vi "EquiRipple Filter Design - DFD.vi"() -> ()   [LabVIEW 2023]
doc: "Demonstrates how to design an Equi-Ripple FIR filter using VIs in the LabVIEW Digital Filter Design Toolkit. \n\nAs you change the Filter Type, experiment with the parameters for that filter type and observe their effect on the magnitude and phase responses."
uses:
  <vilib>/addons/Digital Filter Design/_Objects.llb/DFD Phase Setting.ctl
  <vilib>/addons/Digital Filter Design/Analysis.llb/DFD Plot Freq Response (Linear-Spaced).vi
  <vilib>/addons/Digital Filter Design/NI_DigFilterLicensed.lvlib
panel:
  out "Error message":string
  out "?":string="dB"
  in  "sampling rate":dbl=1000.0 format="%0.2f"
  in  "Display":bool=TRUE
  in  "Bandstop params":T1={"low pass frequency"=100.0, "high pass frequency"=400.0, "low stop frequency"=200.0, "high stop frequency"=300.0} {"high stop frequency" format="%0.2f"; "low stop frequency" format="%0.2f"; "high pass frequency" format="%0.2f"; "low pass frequency" format="%0.2f"}
  in  "Bandpass params":T1={"low pass frequency"=200.0, "high pass frequency"=300.0, "low stop frequency"=100.0, "high stop frequency"=400.0} {"high stop frequency" format="%0.2f"; "low stop frequency" format="%0.2f"; "high pass frequency" format="%0.2f"; "low pass frequency" format="%0.2f"}
  in  "stop":bool
  in  "Highpass params":T2={"stop frequency"=200.0, "pass frequency"=300.0} {"pass frequency" format="%0.2f"; "stop frequency" format="%0.2f"}
  in  "Lowpass params":T3={"pass frequency"=200.0, "stop frequency"=300.0} {"stop frequency" format="%0.2f"; "pass frequency" format="%0.2f"}
  in  "Filter Type":T4(ring)=enum."Bandpass"
  in  "No. of Taps":i32=30
  out "Phase":cluster{"f0":dbl, "df":dbl, "values":dbl[]}[](graph)
  out "Magnitude Response":cluster{"f0":dbl, "df":dbl, "values":dbl[]}[](graph)
  # "Select Help»Show Context Help and move the cursor over the VI icon for more information."
  # "Hz"
  # "radians"
  # "Hz"
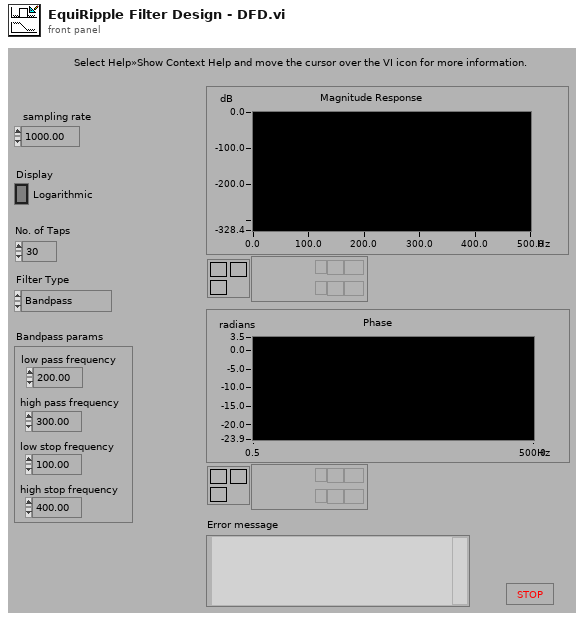
[diagram p1: front panel]
types:
  T1 = cluster{"low pass frequency":dbl, "high pass frequency":dbl, "low stop frequency":dbl, "high stop frequency":dbl}
  T2 = cluster{"stop frequency":dbl, "pass frequency":dbl}
  T3 = cluster{"pass frequency":dbl, "stop frequency":dbl}
  T4 = enum16{"Lowpass", "Highpass", "Bandpass", "Bandstop"}
  T5 = typedef "NI_DigFilterLicensed.lvlib/DFD Phase Setting.ctl" = cluster{"unwrap? (F)":bool, "degree? (F)":bool}
  T6 = cluster{"[0]":bool, "[1]":bool, "[2]":bool, "[3]":bool}
  T7 = cluster{"band specification":cluster{"freq":dbl, "amplitude":dbl, "weight":dbl}[], "ripple constraint":dbl}[]
  T8 = typedef "NI_DigFilterLicensed.lvlib/DFD Filter Obj.ctl" = cluster{"mSRate_Fs":dbl, "mSRate_Version":string, "mSRate_Comments":string, "mSRate_OrgCoef":T9, "mSRate_CurCoef":T9, "mSRate_Quantized?":bool, "mSRate_QCoef":T9, "mSRate_QSettings":T11[], "mSRate_Order":i32, "mSRate_Scaling":cluster{"mSRate_ScaleByPowerOf2?":bool, "mSRate_ScaleType":T13}}
  T9 = typedef "NI_DigFilterLicensed.lvlib/DFD Filter Coef.ctl" = cluster{"type":T10, "gain":dbl, "coef a (k)":dbl[], "coef b (v)":dbl[]}
  T10 = typedef "NI_DigFilterLicensed.lvlib/DFD Filter Structure Type Selector.ctl" = enum16{"Undefined", "FIR Direct Form", "FIR Direct Form Transposed", "FIR Symmetric", "FIR Antisymmetric", "IIR Direct Form I", "IIR Direct Form I Transposed", "IIR Direct Form II", "IIR Direct Form II Transposed", "IIR Cascaded Second Order Sections Form I", "IIR Cascaded Second Order Sections Form I Transposed", "IIR Cascaded Second Order Sections Form II", "IIR Cascaded Second Order Sections Form II Transposed", "Lattice Allpass (basic sections)", "Lattice Allpass (one multiplier sections)", "Lattice Allpass (normalized sections)", "Lattice AR (basic sections)", "Lattice AR (one multiplier sections)", "Lattice AR (normalized sections)", "Lattice MA (minimum phase)", "Lattice MA (maximum phase)", "Lattice ARMA (basic sections)", "Lattice ARMA (one multiplier sections)", "Lattice ARMA (normalized sections)"}
  T11 = typedef "NI_DigFilterLicensed.lvlib/dfd_Internal Quantization Settings.ctl" = cluster{"source":T12, "wl":i16, "iwl":i16, "overflow mode":enum16{"Saturation", "Wrap"}, "rounding mode":enum16{"Nearest", "Truncation"}, "signed?":bool}
  T12 = typedef "NI_DigFilterLicensed.lvlib/dfd_Internal Quantization Srcs.ctl" = u16
  T13 = typedef "NI_DigFilterLicensed.lvlib/DFD Coef Norm Type.ctl" = enum16{"No Norm", "Time Domain 1-Norm", "Time Domain 2-Norm", "Time Domain Inf-Norm"}
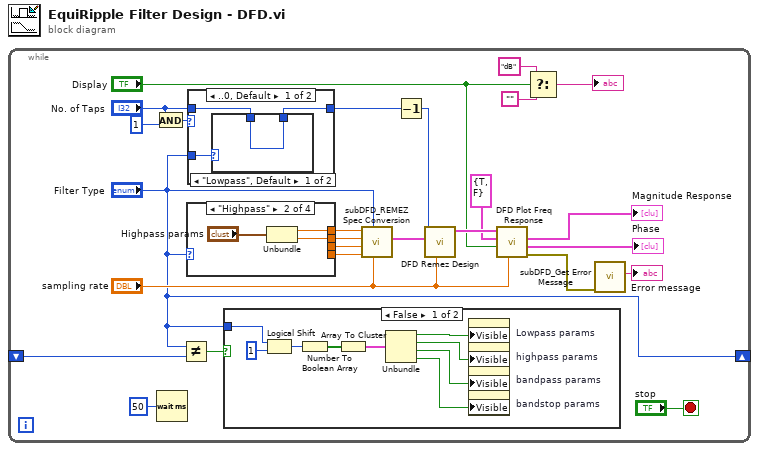
[diagram p0: block diagram]
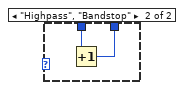
[diagram p2: hidden frame]
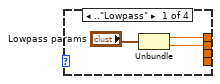
[diagram p5: hidden frame]
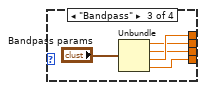
[diagram p6: hidden frame]
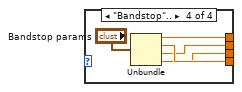
[diagram p7: hidden frame]
diagram:
  n1 = while {
    shift-left: _ -> [w26]
    shift-right: ["Filter Type"] -> _
    stop <- "stop" stop-if-true
    n2 = And(x="No. of Taps", y=1) -> (x .and. y?=w7:i32)
    n3 = Wait (ms)(milliseconds to wait=u32 50) -> ()  [unwired: 1 out]
    n4 = Not Equal?(x="Filter Type", y=w26) -> (x != y?=w25:bool)
    n5 = case shown="\"Highpass\"" "Filter Type" {
      tunnel: [w45 w47 w52 w57] -> w23
      tunnel: [w44 w46 w51 w55] -> w22
      tunnel: [_ _ w50 w54] -> w21
      tunnel: [_ _ w49 w56] -> w20
      frame .."Lowpass" {
        n6 = Unbundle("Lowpass params") -> ("pass frequency"=w45:dbl, "stop frequency"=w44:dbl)
      }
      frame "Highpass" {
        n7 = Unbundle("Highpass params") -> ("stop frequency"=w47:dbl, "pass frequency"=w46:dbl)
      }
      frame "Bandpass" {
        n8 = Unbundle("Bandpass params") -> ("low pass frequency"=w51:dbl, "high pass frequency"=w50:dbl, "low stop frequency"=w52:dbl, "high stop frequency"=w49:dbl)
      }
      frame "Bandstop".. {
        n9 = Unbundle("Bandstop params") -> ("low pass frequency"=w57:dbl, "high pass frequency"=w56:dbl, "low stop frequency"=w55:dbl, "high stop frequency"=w54:dbl)
      }
    }
    n10 = case shown="..0, Default" w7 {
      tunnel: "No. of Taps" -> [w28 w33]
      tunnel: [w27 w33] -> w5
      tunnel: "Filter Type" -> [w29 _]
      frame ..0, Default {
        n11 = case shown="\"Lowpass\", Default" w29 {
          tunnel: w28 -> [w30 w32]
          tunnel: [w30 w31] -> w27
          frame "Lowpass", Default {
          }
          frame "Highpass", "Bandstop" {
            n12 = Increment(x=w32) -> (x+1=w31:i32)
          }
        }
      }
      frame 1.. {
      }
    }
    n13 = case shown="False" w25 {
      tunnel: "Filter Type" -> [w42 _]
      frame False {
        n14 = Logical Shift(y=w42, x=1) -> (x << y=w40:i32)
        n15 = Number To Boolean Array(number=w40) -> (Boolean array=w39:bool[])
        n16 = Array To Cluster(array=w39) -> (cluster=w38:T6)
        n17 = Unbundle(w38) -> ("[0]"=w37:bool, "[1]"=w36:bool, "[2]"=w35:bool, "[3]"=w34:bool)
        n18 = property on="Lowpass params" class="Clust (strict)"("Visible"=w37) -> ()  [unwired: 2 in, 2 out]
        n19 = property on="highpass params" class="Clust (strict)"("Visible"=w36) -> ()  [unwired: 2 in, 2 out]
        n20 = property on="bandpass params" class="Clust (strict)"("Visible"=w35) -> ()  [unwired: 2 in, 2 out]
        n21 = property on="bandstop params" class="Clust (strict)"("Visible"=w34) -> ()  [unwired: 2 in, 2 out]
      }
      frame True {
      }
    }
    n22 = call "subDFD_REMEZ Spec Conversion.vi"("fs [Hz]"="sampling rate", "Filter Type"="Filter Type", "f4 [Hz]"=w20, "f3 [Hz]"=w21, "f2 [Hz]"=w22, "f1 [Hz]"=w23) -> ("band specs"=w19:T7)  [unwired: 5 out]
    n23 = Decrement(x=w5) -> (x-1=w15:i32)
    n24 = call <vilib>:"DFD Remez Design.vi"("fs [Hz]"="sampling rate", "band specs"=w19, "order"=w15) -> ("filter out"=w14:T8)  [unwired: 4 in, 4 out]
    n25 = call-poly <vilib>:"DFD Plot Freq Response.vi"("fs [Hz]"="sampling rate", "dB on? (T)"="Display", "phase view"=T5 {"unwrap? (F)"=TRUE, "degree? (F)"=FALSE}, "filter in"=w14) -> ("error out"=w2:errorcluster, "phase response"=→"Phase":cluster{"f0":dbl, "df":dbl, "values":dbl[]}[], "magnitude response"=→"Magnitude Response":cluster{"f0":dbl, "df":dbl, "values":dbl[]}[])  [unwired: 4 in, 1 out]
    n26 = Select(t="dB", s="Display", f="") -> (s? t:f=→"?":string)
    n27 = call <vilib>:"subDFD_Get Error Message.vi"("error in (no error)"=w2) -> ("Error Message"=→"Error message":string)  [unwired: 10 out]
  }
